vi "Launch Nested Actors.vi"(8 "error in (no error)":errorcluster, 11 "Elevator Controller Actor in":refnum<class "Elevator Controller Actor.lvclass">) -> (0 "error out":errorcluster, 3 "Elevator Controller Actor out":refnum<class "Elevator Controller Actor.lvclass">)   [LabVIEW 2022 SP3, in "Elevator Controller Actor.lvlib" / "Elevator Controller Actor.lvclass"]
uses:
  Elevator Controller Actor.lvclass
  Elevator Controller Actor.lvclass/Elevator Controller Actor.ctl
  <vilib>/ActorFramework/Actor/Actor.lvclass
  C:/Program Files/National Instruments/LabVIEW 2022/vi.lib/ActorFramework/Actor/Actor.lvclass
  C:/Workspace/CLA/Elevator AF_2022_2nd/Elevator Controller Actor/Elevator Controller Actor/Elevator Controller Actor.lvclass
  C:/Workspace/CLA/Elevator AF_2022_2nd/Interface 3/Interface 3.lvclass
  Sim User Console Actor/Elevator Controller Actor/Sim User Console Actor.lvclass
  Sim Display Console Actor/Elevator Controller Actor/Sim Display Console Actor.lvclass
  Sim Sensor Interface Actor/Elevator Controller Actor/Sim Sensor Interface Actor.lvclass
  Configuration Database Actor/Configuration Database Actor/Configuration Database Actor.lvclass
  C:/Workspace/CLA/Elevator AF_2022_2nd/User Console Actor/User Console Actor/User Console Actor.lvclass
  C:/Workspace/CLA/Elevator AF_2022_2nd/Sim User Console Actor/Elevator Controller Actor/Sim User Console Actor.lvclass
  C:/Workspace/CLA/Elevator AF_2022_2nd/Display Console Actor/Display Console Actor/Display Console Actor.lvclass
  C:/Workspace/CLA/Elevator AF_2022_2nd/Sim Display Console Actor/Elevator Controller Actor/Sim Display Console Actor.lvclass
  C:/Workspace/CLA/Elevator AF_2022_2nd/Sensor Interface Actor/Sensor Interface Actor/Sensor Interface Actor.lvclass
  C:/Workspace/CLA/Elevator AF_2022_2nd/Sim Sensor Interface Actor/Elevator Controller Actor/Sim Sensor Interface Actor.lvclass
  C:/Workspace/CLA/Elevator AF_2022_2nd/Configuration Database Actor/Configuration Database Actor/Configuration Database Actor.lvclass
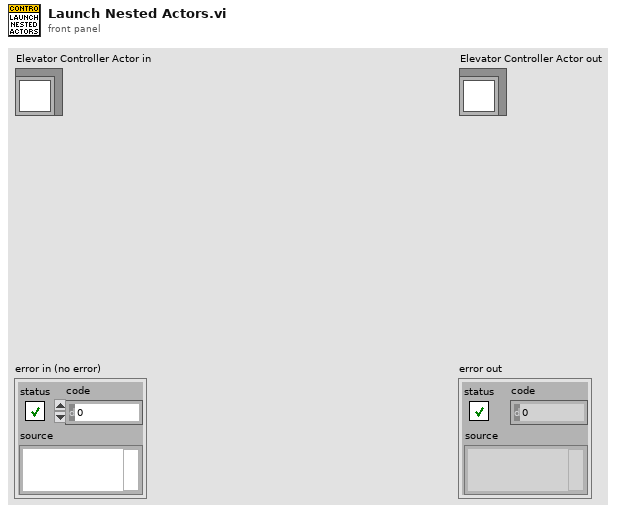
[diagram p1: front panel]
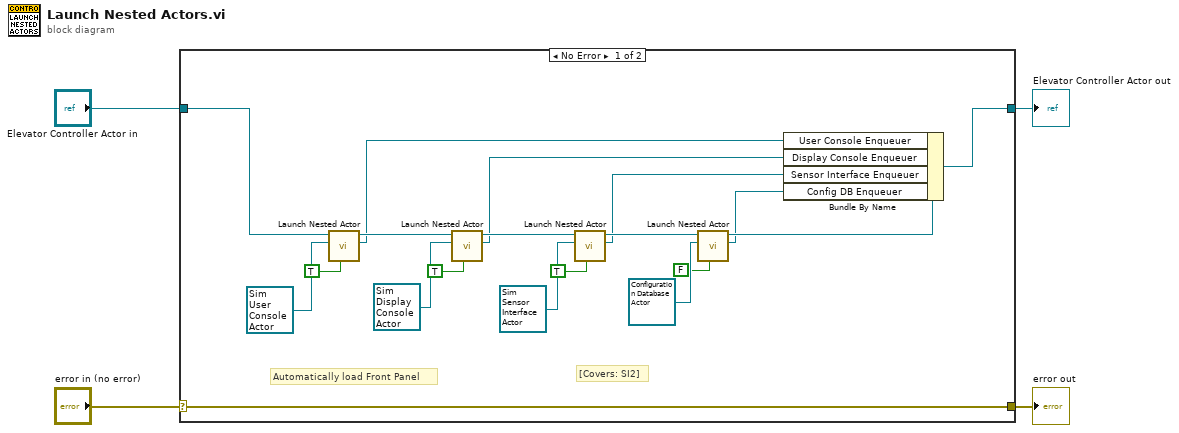
[diagram p0: block diagram]
diagram:
  n1 = case shown="No Error" "error in (no error)" {
    selector: "error in (no error)" -> [w23 w25]
    tunnel: [w23 w25] -> w3
    tunnel: [w18 w24] -> w1
    tunnel: "Elevator Controller Actor in" -> [w19 w24]
    frame No Error {
      # "Automatically load Front Panel"
      # "[Covers: SI2]"
      n2 = call <vilib>:"Launch Nested Actor.vi"("Open Actor Core front panel? (F)"=TRUE, "Nested Actor"=refnum<class "Sim User Console Actor.lvclass"> refnum ("Sim User Console Actor.lvlib:Sim User Console Actor.lvclass"), "Caller Actor in"=w19) -> ("Nested Actor's Enqueuer"=w12:refnum<class "Message Enqueuer.lvclass">, "Caller Actor out"=w22:refnum<class "Elevator Controller Actor.lvclass">)  [unwired: 6 in, 1 out]
      n3 = call <vilib>:"Launch Nested Actor.vi"("Open Actor Core front panel? (F)"=TRUE, "Nested Actor"=refnum<class "Sim Display Console Actor.lvclass"> refnum ("Sim Display Console Actor.lvlib:Sim Display Console Actor.lvclass"), "Caller Actor in"=w22) -> ("Nested Actor's Enqueuer"=w11:refnum<class "Message Enqueuer.lvclass">, "Caller Actor out"=w21:refnum<class "Elevator Controller Actor.lvclass">)  [unwired: 6 in, 1 out]
      n4 = call <vilib>:"Launch Nested Actor.vi"("Open Actor Core front panel? (F)"=TRUE, "Nested Actor"=refnum<class "Sim Sensor Interface Actor.lvclass"> refnum ("Sim Sensor Interface Actor.lvlib:Sim Sensor Interface Actor.lvclass"), "Caller Actor in"=w21) -> ("Nested Actor's Enqueuer"=w10:refnum<class "Message Enqueuer.lvclass">, "Caller Actor out"=w20:refnum<class "Elevator Controller Actor.lvclass">)  [unwired: 6 in, 1 out]
      n5 = call <vilib>:"Launch Nested Actor.vi"("Open Actor Core front panel? (F)"=FALSE, "Nested Actor"=refnum<class "Configuration Database Actor.lvclass"> refnum ("Configuration Database Actor.lvlib:Configuration Database Actor.lvclass"), "Caller Actor in"=w20) -> ("Nested Actor's Enqueuer"=w9:refnum<class "Message Enqueuer.lvclass">, "Caller Actor out"=w17:refnum<class "Elevator Controller Actor.lvclass">)  [unwired: 6 in, 1 out]
      n6 = Bundle By Name(cluster=w17, "User Console Enqueuer"=w12, "Display Console Enqueuer"=w11, "Sensor Interface Enqueuer"=w10, "Config DB Enqueuer"=w9) -> (w18:refnum<class "Elevator Controller Actor.lvclass">)
    }
    frame Error {
    }
  }
  "error out" <- w3
  "Elevator Controller Actor out" <- w1
